vi "Update_Current_Value_client.vi"(0 "Don't Bother with check?":bool, 1 "Update array in":T1[](array[typedef]) {"New Value" format="%.2f"}) -> ()   [LabVIEW 2021]
doc: "This is an example of using features of the VI Server as a client. It shows how you might browse from one or more applications that may be exporting data from one or more data stations. \n\nThe example shows how to query a server for its list of exported VIs, how to get references to the VIs, and how call them with the Call By Reference function."
uses:
  Sub VIs/ADAM Controls/Update_scan_value.ctl
  Anemometry/Anemometry Sub Vis/Controls/Global_mode.ctl
  Anemometry/Anemometry Sub Vis/Globals/Preference_global.vi
panel:
  in  "Server type":refnum<vi>
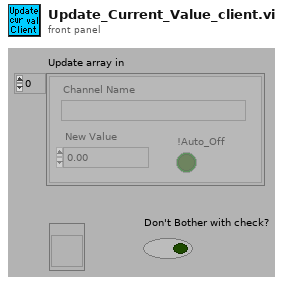
[diagram p1: front panel]
types:
  T1 = typedef "Update_scan_value.ctl" = cluster{"Channel Name":string, "New Value":dbl, "!Auto_Off":bool}
  T2 = typedef "Server_Comms.ctl" = enum16{"Do Not Link To Server", "Server Link Healthy"}
  T3 = typedef "Global_mode.ctl" = enum16{"Read Global", "Load Global From File", "Write Global to File"}
  T4 = enum16{"Append to Global", "Read Global then Clear"}
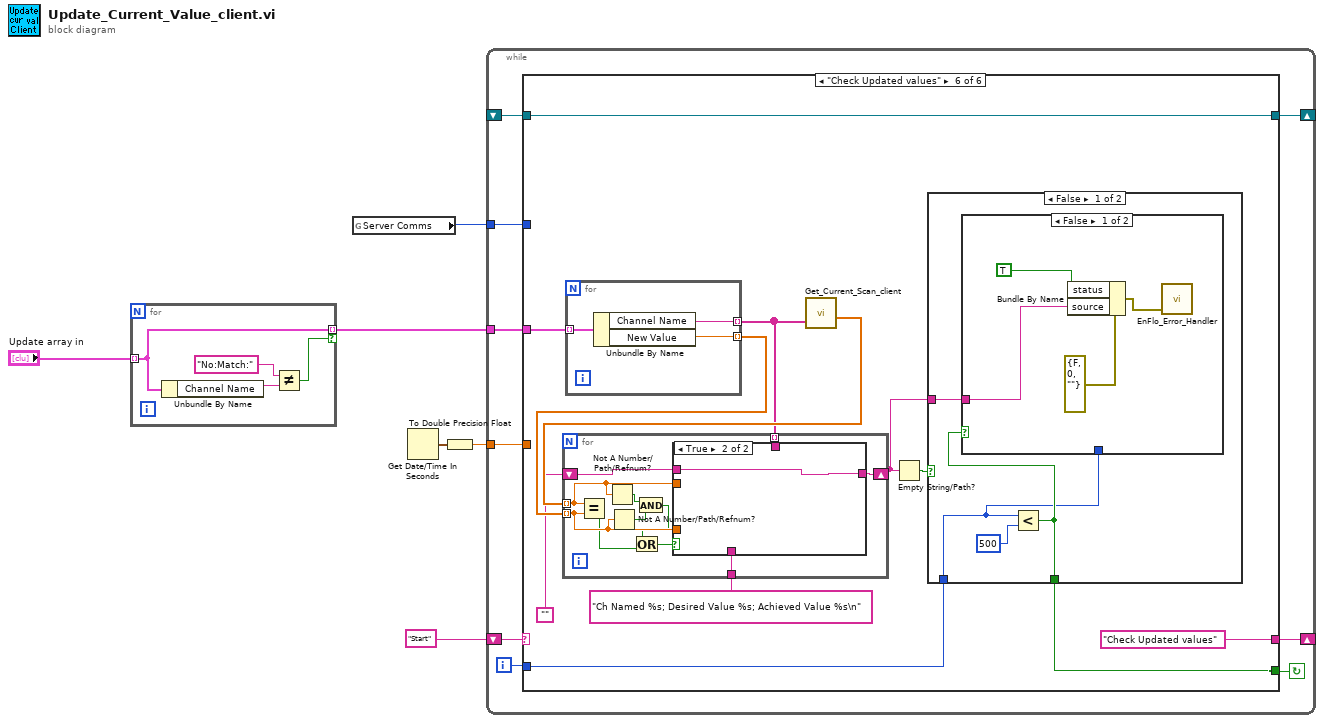
[diagram p0: block diagram]
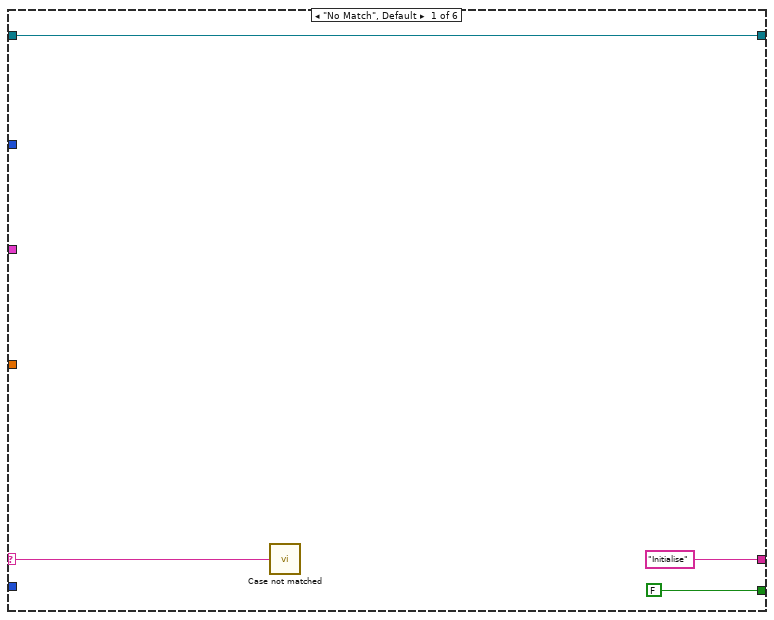
[diagram p2: hidden frame]
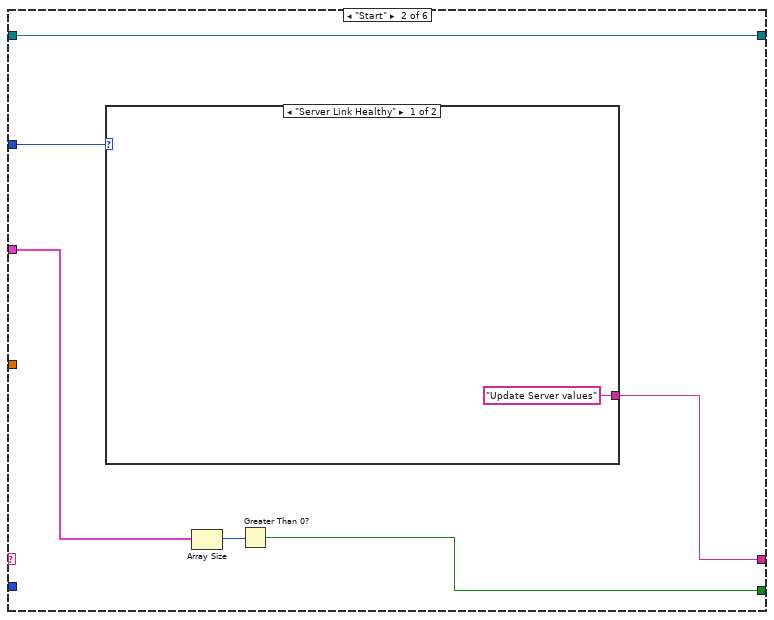
[diagram p3: hidden frame]
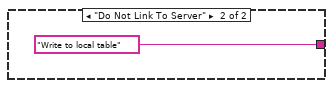
[diagram p4: hidden frame]
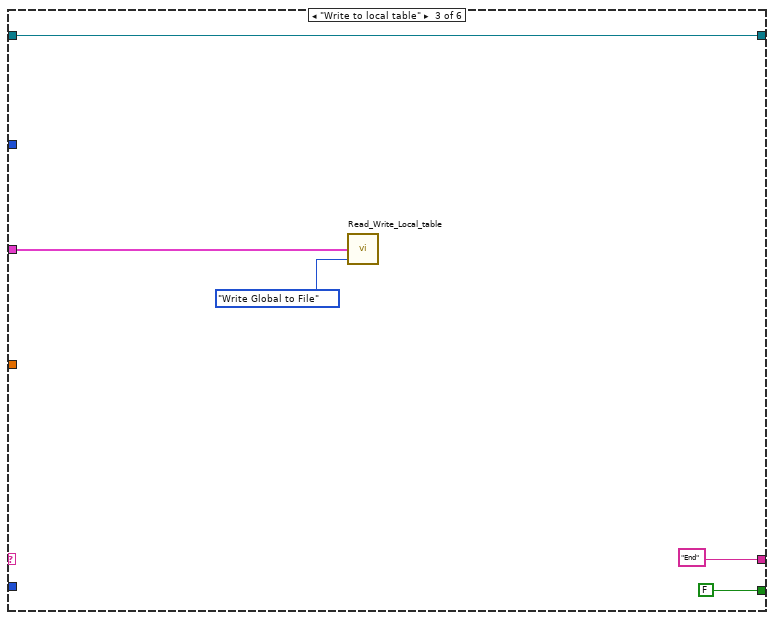
[diagram p5: hidden frame]
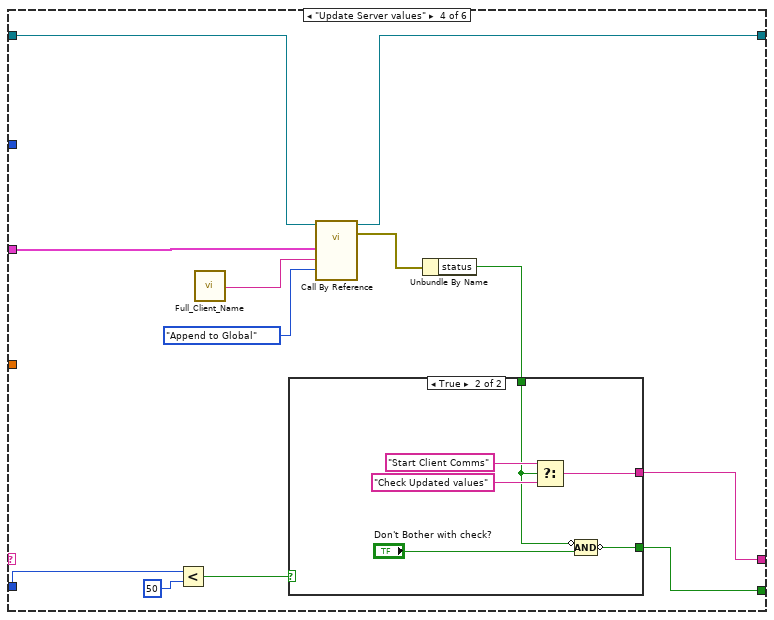
[diagram p6: hidden frame]
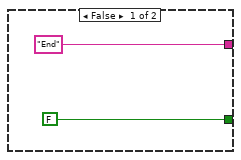
[diagram p7: hidden frame]
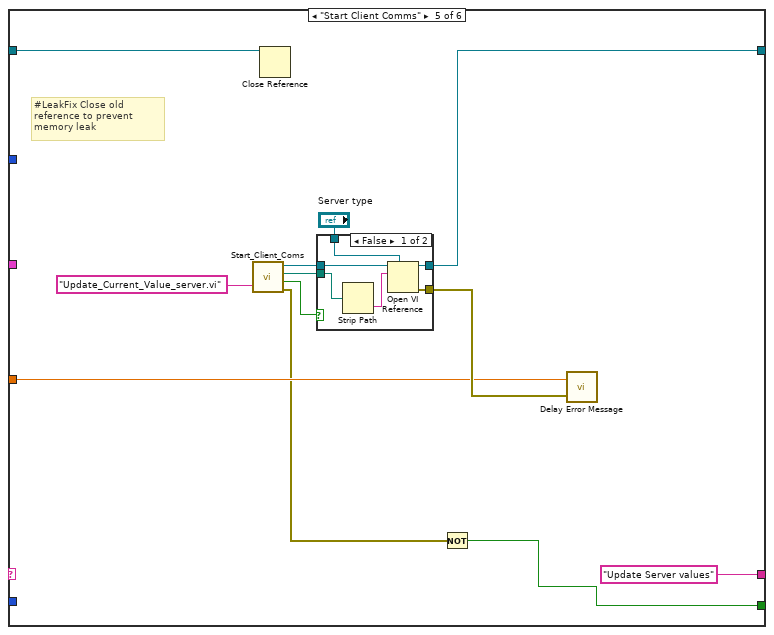
[diagram p8: hidden frame]
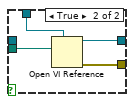
[diagram p9: hidden frame]
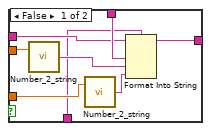
[diagram p10: hidden frame]
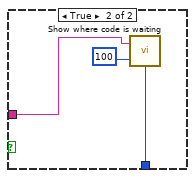
[diagram p11: hidden frame]
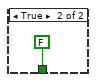
[diagram p12: hidden frame]
diagram:
  n1 = for {
    tunnel: "Update array in" -> [w8] mode=indexing
    tunnel: [w8] -> w1 mode=indexing if=w7
    n2 = Unbundle By Name(w8) -> ("Channel Name"=w10:string)
    n3 = Not Equal?(x="No:Match:", y=w10) -> (x != y?=w7:bool)
  }
  n4 = global read "Preference_global.vi" "Server Comms"() -> (w5:T2)
  n5 = Get Date/Time In Seconds() -> (seconds since 1Jan1904=w4:timestamp)
  n6 = To Double Precision Float(number=w4) -> (double precision float=w3:dbl)
  n7 = while {
    shift-left: "Start" -> [w17]
    shift-right: [w18] -> _
    tunnel: w5 -> [w16]
    tunnel: w1 -> [w15]
    shift-right: [w13] -> _
    shift-left: _ -> [w14]
    tunnel: w3 -> [w11]
    i -> [w12]
    stop <- w19 continue-if-true
    n8 = case shown="\"Check Updated values\"" w17 {
      selector: w17 -> [w20 _ _ _ _ _]
      tunnel: [FALSE w25 FALSE w37 w57 w88] -> w19
      tunnel: ["Initialise" w24 "End" w42 "Update Server values" "Check Updated values"] -> w18
      tunnel: w16 -> [_ w29 _ _ _ _]
      tunnel: w15 -> [_ w27 w33 w46 _ w90]
      tunnel: w14 -> [w21 w28 w32 w44 w61 w89]
      tunnel: [w21 w28 w32 w45 w63 w89] -> w13
      tunnel: w12 -> [_ _ _ w40 _ w79]
      tunnel: w11 -> [_ _ _ _ w59 _]
      frame "No Match", Default {
        n9 = call "Case not matched.vi"("Case Name not Matched"=w20) -> ()
      }
      frame "Start" {
        n10 = case shown="\"Server Link Healthy\"" w29 {
          tunnel: ["Update Server values" "Write to local table"] -> w24
          frame "Server Link Healthy" {
          }
          frame "Do Not Link To Server" {
          }
        }
        n11 = Array Size(array=w27) -> (size(s)=w26:i32)
        n12 = Greater Than 0?(x=w26) -> (x > 0?=w25:bool)
      }
      frame "Write to local table" {
        n13 = call "Read_Write_Local_table.vi"("Mode"=Global_mode."Write Global to File", "Ch Values in"=w33) -> ()  [unwired: 1 in, 3 out]
      }
      frame "Update Server values" {
        n14 = Less?(x=w40, y=50) -> (x < y?=w38:bool)
        n15 = call "Full_Client_Name.vi"() -> ("Client Name"=w48:string)
        n16 = call-by-ref "?"(reference=w44, "Mode"=T4."Append to Global", "Client HD name"=w48, "Update array in"=w46) -> (reference out=w45:refnum<vi>, error out=w41:errorcluster)  [unwired: 1 in, 1 out]
        n17 = Unbundle By Name(w41) -> ("status"=w43:bool)
        n18 = case shown="True" w38 {
          tunnel: w43 -> [_ w53]
          tunnel: ["End" w54] -> w42
          tunnel: [FALSE w51] -> w37
          frame False {
          }
          frame True {
            n19 = Select(t="Start Client Comms", s=w53, f="Check Updated values") -> (s? t:f=w54:string)
            n20 = Compound Arithmetic op=AND(invert w53, "Don't Bother with check?") -> (invert w51:bool)
          }
        }
      }
      frame "Start Client Comms" {
        # "#LeakFix Close old reference to prevent memory leak"
        n21 = call "Start_Client_Coms.vi"("VI name to run on server"="Update_Current_Value_server.vi") -> ("LabVIEW application reference"=w66:refnum<vi>, "Checked VI name"=w65:path, "Local Call"=w67:bool, "Error cluster"=w58:errorcluster)  [unwired: 1 in]
        n22 = Close Reference(reference=w61) -> ()  [unwired: 1 in, 1 out]
        n23 = case shown="False" w67 {
          tunnel: [w73 w78] -> w63
          tunnel: "Server type" -> [w71 w77]
          tunnel: w65 -> [w70 w76]
          tunnel: w66 -> [w69 _]
          tunnel: [w72 w75] -> w60
          frame False {
            n24 = Strip Path(path=w70) -> (name=w74:string)  [unwired: 1 out]
            n25 = Open VI Reference(type specifier VI Refnum (for type only)=w71, application reference (local)=w69, vi path=w74) -> (vi reference=w73:refnum<vi>, error out=w72:errorcluster)  [unwired: 1 in, 2 out]
          }
          frame True {
            n26 = Open VI Reference(type specifier VI Refnum (for type only)=w77, vi path=w76) -> (vi reference=w78:refnum<vi>, error out=w75:errorcluster)  [unwired: 1 in, 3 out]
          }
        }
        n27 = Not(x=w58) -> (.not. x?=w57:bool)
        n28 = call "Delay Error Message.vi"("error in (no error)"=w60, "Seconds since 1904"=w59) -> ()  [unwired: 2 in]
      }
      frame "Check Updated values" {
        n29 = for {
          tunnel: w90 -> [w125] mode=indexing
          tunnel: [w124] -> w84 mode=indexing
          tunnel: [w123] -> w86 mode=indexing
          n30 = Unbundle By Name(w125) -> ("Channel Name"=w124:string, "New Value"=w123:dbl)
        }
        n31 = call "Get_Current_Scan_client.vi"("multipleChannels"=w84) -> ("Numerical Values"=w85:dbl[])  [unwired: 1 in, 3 out]
        n32 = for {
          shift-right: [w99] -> w80
          shift-left: "" -> [w98]
          tunnel: w86 -> [w95] mode=indexing
          tunnel: w85 -> [w96] mode=indexing
          tunnel: w84 -> [w101] mode=indexing
          tunnel: "Ch Named %s; Desired Value %s; Achieved Value %s\n" ("format string") -> [w100]
          n33 = Equal?(x=w96, y=w95) -> (x = y?=w91:bool)
          n34 = Not A Number/Path/Refnum?(number/path/refnum=w96) -> (NaN/Path/Refnum?=w93:bool)
          n35 = Not A Number/Path/Refnum?(number/path/refnum=w95) -> (NaN/Path/Refnum?=w94:bool)
          n36 = And(x=w93, y=w94) -> (x .and. y?=w92:bool)
          n37 = Or(x=w92, y=w91) -> (x .or. y?=w97:bool)
          n38 = case shown="True" w97 {
            tunnel: w101 -> [w109 _]
            tunnel: w96 -> [w103 _]
            tunnel: w95 -> [w104 _]
            tunnel: w100 -> [w102 _]
            tunnel: [w108 w110] -> w99
            tunnel: w98 -> [w107 w110]
            frame False {
              n39 = call "Number_2_string.vi"("number"=w103) -> ("String"=w105:string)  [unwired: 1 in]
              n40 = call "Number_2_string.vi"("number"=w104) -> ("String"=w106:string)  [unwired: 1 in]
              n41 = Format Into String(format string=w102, initial string=w107, w109, w105, w106) -> (resulting string=w108:string)  [unwired: 1 in, 1 out]
            }
            frame True {
            }
          }
        }
        n42 = Empty String/Path?(string/path=w80) -> (empty?=w81:bool)
        n43 = case shown="False" w81 {
          tunnel: [w112 FALSE] -> w88
          tunnel: w80 -> [w114 _]
          tunnel: w79 -> [w111 _]
          frame False {
            n44 = Less?(x=w111, y=500) -> (x < y?=w112:bool)
            n45 = case shown="False" w112 {
              tunnel: w114 -> [w117 w120]
              tunnel: w111 -> [_ w119]
              frame False {
                n46 = Bundle By Name(cluster=errorcluster {"status"=FALSE, "code"=0, "source"=""} ("error in (no error)"), "status"=TRUE, "source"=w117) -> (w115:errorcluster)
                n47 = call "EnFlo_Error_Handler.vi"("error in (no error)"=w115) -> ()  [unwired: 2 in, 3 out]
              }
              frame True {
                n48 = call "Show where code is waiting.vi"("Loop index"=w119, "Wait (ms)"=u32 100 ("milliseconds to wait"), "Message"=w120) -> ()  [unwired: 1 in]
              }
            }
          }
          frame True {
          }
        }
      }
    }
  }
